vi "UDP Data Link - Configuration Utilities - Remove Old Rx Channels.vi"(8 "error in (no error)":errorcluster, 11 "Device Item Ref in":T1 format="%.0x") -> (0 "error out":errorcluster, 2 "Rx Dependent Refs":T1[](array[typedef]) format="%.0x", 3 "Device Item Ref out":T1 format="%.0x")   [LabVIEW 2015, in "UDP-Custom-Device System Explorer.lvlib"]
uses:
  UDP-Custom-Device System Explorer.lvlib
  <vilib>/NI Veristand/Custom Device API/Custom Device Item Ref.ctl
  Shared/Constants.vi
  <vilib>/NI Veristand/Custom Device Tools/Custom Device Utility Library/NI VeriStand - Search for Item by GUID.vi
  <vilib>/NI Veristand/Custom Device API/Get Item Property (String Array).vi
  <vilib>/NI Veristand/Custom Device API/Set Item Property (String Array).vi
  <vilib>/NI VeriStand/Custom Device Tools/Custom Device Utility Library/Custom Device Utility Library.lvlib
  <vilib>/NI VeriStand/Custom Device API/Custom Device API.lvlib
  Shared/UDP-Custom-Device Shared.lvlib
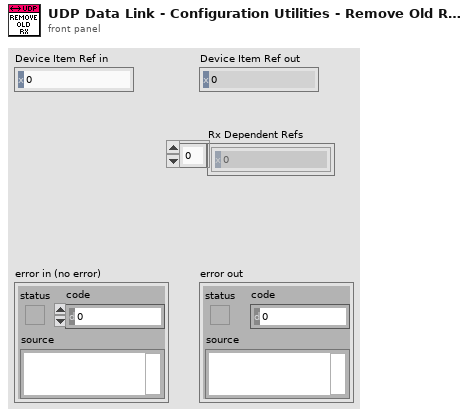
[diagram p1: front panel]
types:
  T1 = typedef "Custom Device API.lvlib/Custom Device Item Ref.ctl" = u64
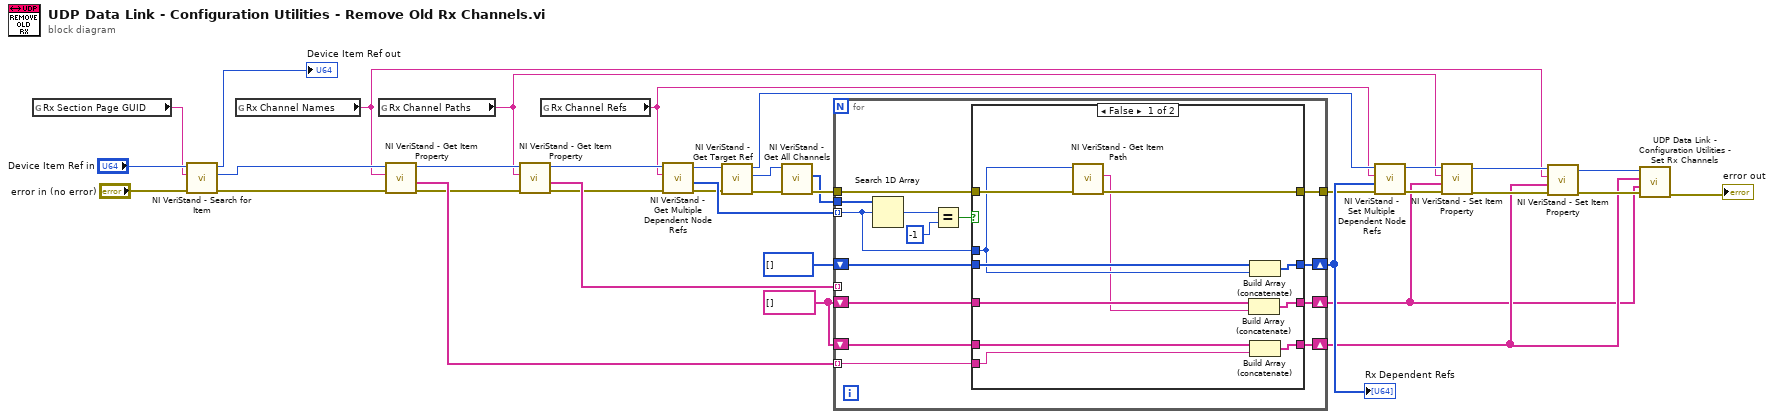
[diagram p0: block diagram]
diagram:
  w27 = string[] []
  n1 = global read "Constants.vi" "Rx Section Page GUID"() -> (w3:string)
  n2 = call-poly <vilib>:"NI VeriStand - Search for Item.vi"("error in"="error in (no error)", "Item GUID"=w3, "Section Ref in"="Device Item Ref in") -> ("error out"=w19:errorcluster, "Item Ref"=w21:T1, "Section Ref out"=→"Device Item Ref out":T1)  [unwired: 5 in, 1 out]
  n3 = global read "Constants.vi" "Rx Channel Names"() -> (w4:string)
  n4 = global read "Constants.vi" "Rx Channel Paths"() -> (w1:string)
  n5 = call-poly <vilib>:"NI VeriStand - Get Item Property.vi"("error in (no error)"=w19, "Property Name"=w4, "Item Ref in"=w21) -> ("error out"=w20:errorcluster, "Value"=w25:string[], "Item Ref out"=w22:T1)  [unwired: 5 in, 1 out]
  n6 = call-poly <vilib>:"NI VeriStand - Get Item Property.vi"("error in (no error)"=w20, "Property Name"=w1, "Item Ref in"=w22) -> ("error out"=w24:errorcluster, "Value"=w26:string[], "Item Ref out"=w23:T1)  [unwired: 5 in, 1 out]
  n7 = global read "Constants.vi" "Rx Channel Refs"() -> (w2:string)
  n8 = call <vilib>:"NI VeriStand - Get Multiple Dependent Node Refs.vi"("error in (no error)"=w24, "Base Property Name"=w2, "Item Ref in"=w23) -> ("error out"=w12:errorcluster, "Dependent Node Refs"=w17:T1[], "Item Ref out"=w14:T1)  [unwired: 6 in]
  n9 = call <vilib>:"NI VeriStand - Get Target Ref.vi"("error in"=w12, "Item Ref in"=w14) -> ("error out"=w13:errorcluster, "Target Ref"=w15:T1, "Item Ref out"=w30:T1)  [unwired: 6 in, 1 out]
  n10 = call <vilib>:"NI VeriStand - Get All Channels.vi"("error in"=w13, "Section Ref in"=w15) -> ("error out"=w18:errorcluster, "Channel Refs"=w16:T1[])  [unwired: 6 in, 2 out]
  n11 = for {
    tunnel: w16 -> [w50]
    tunnel: w17 -> [w38] mode=indexing
    tunnel: w18 -> [w46]
    tunnel: w25 -> [w45] mode=indexing
    tunnel: w26 -> [_] mode=indexing
    shift-right: [w40] -> w6
    shift-left: w27 -> [w43]
    shift-right: [w39] -> w7
    shift-left: w27 -> [w44]
    shift-right: [w41] -> w31
    shift-left: T1[] [] -> [w42]
    tunnel: [w37] -> w29
    n12 = Search 1D Array(1D array=w50, element=w38) -> (index of element=w49:i32)  [unwired: 1 in]
    n13 = Equal?(x=w49, y=-1) -> (x = y?=w47:bool)
    n14 = case shown="False" w47 {
      tunnel: w46 -> [w54 w62]
      tunnel: w45 -> [w56 _]
      tunnel: w44 -> [w57 w63]
      tunnel: w43 -> [w59 w64]
      tunnel: w42 -> [w61 w65]
      tunnel: [w60 w65] -> w41
      tunnel: [w58 w64] -> w40
      tunnel: [w55 w63] -> w39
      tunnel: w38 -> [w53 _]
      tunnel: [w52 w62] -> w37
      frame False {
        n15 = call <vilib>:"NI VeriStand - Get Item Path.vi"("error in (no error)"=w54, "Item Ref in"=w53) -> ("error out"=w52:errorcluster, "Path"=w51:string)  [unwired: 6 in, 2 out]
        n16 = Build Array (concatenate)(w59, w51) -> (w58:string[])
        n17 = Build Array (concatenate)(w61, w53) -> (w60:T1[])
        n18 = Build Array (concatenate)(w57, w56) -> (w55:string[])
      }
      frame True {
      }
    }
  }
  "Rx Dependent Refs" <- w31
  n19 = call <vilib>:"NI VeriStand - Set Multiple Dependent Node Refs.vi"("error in (no error)"=w29, "Dependent Node Refs"=w31, "Base Property Name"=w2, "Item Ref in"=w30) -> ("error out"=w32:errorcluster, "Item Ref out"=w33:T1)  [unwired: 6 in]
  n20 = call-poly <vilib>:"NI VeriStand - Set Item Property.vi"("error in (no error)"=w32, "Value"=w6, "Property Name"=w1, "Item Ref in"=w33) -> ("error out"=w34:errorcluster, "Item Ref out"=w35:T1)  [unwired: 5 in, 1 out]
  n21 = call-poly <vilib>:"NI VeriStand - Set Item Property.vi"("error in (no error)"=w34, "Value"=w7, "Property Name"=w4, "Item Ref in"=w35) -> ("error out"=w9:errorcluster, "Item Ref out"=w8:T1)  [unwired: 5 in, 1 out]
  n22 = call "UDP Data Link - Configuration Utilities - Set Rx Channels.vi"("error in (no error)"=w9, "Rx Channel Paths"=w6, "Rx Channel Names"=w7, "Item Ref in"=w8) -> ("error out"=→"error out":errorcluster)  [unwired: 6 in, 1 out]
